vi "demark PXI-8431.vi"(8 "error In":errorcluster, 10 "Slot":i32=6) -> (0 "error out":errorcluster, 1 "COM name":string[](array[string]), 2 "VISA Ref":refnum<visa-resource-name>[](array[refnum]))   [LabVIEW 2017]
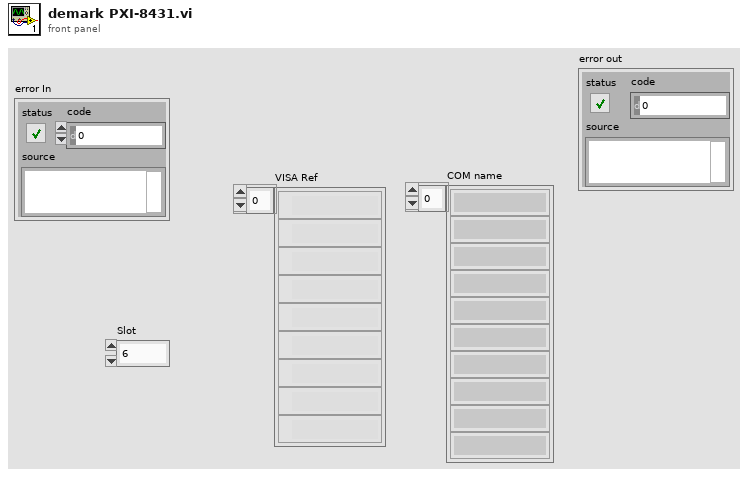
[diagram p1: front panel]
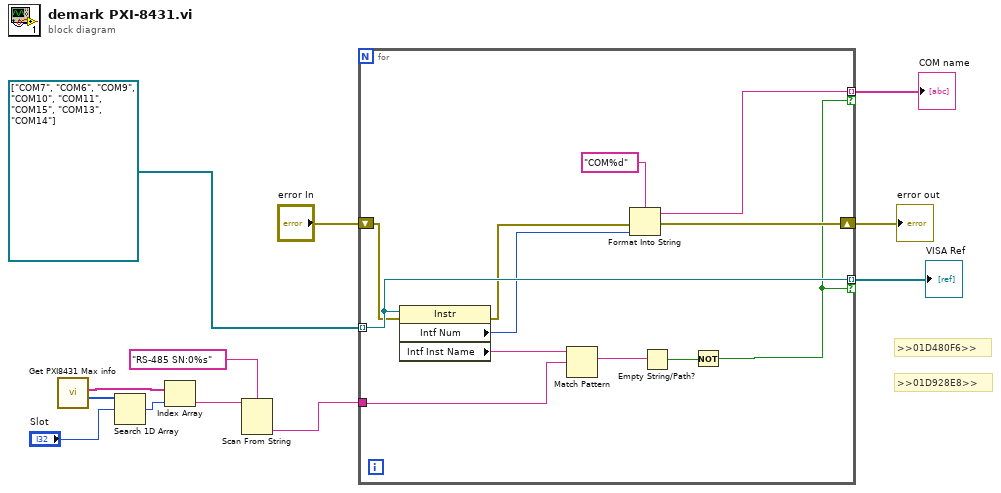
[diagram p0: block diagram]
diagram:
  # ">>01D480F6>>"
  # ">>01D928E8>>"
  n1 = call "Get PXI8431 Max info.vi"() -> ("Slot number"=w7:i32[], "Alias"=w5:string[])  [unwired: 10 in]
  n2 = Search 1D Array(1D array=w7, element="Slot") -> (index of element=w4:i32)  [unwired: 1 in]
  n3 = Index Array(array=w5, index=w4) -> (element=w3:string)
  n4 = Scan From String(format string="RS-485 SN:0%s", input string=w3) -> (output 1=w1:string)  [unwired: 3 in, 3 out]
  n5 = for {
    tunnel: refnum<visa-resource-name>[] ["COM7", "COM6", "COM9", "COM10", "COM11", "COM15", "COM13", "COM14"] -> [w24] mode=indexing
    tunnel: [w24] -> w11 mode=indexing if=w13
    tunnel: [w20] -> w8 mode=indexing if=w13
    shift-right: [w22] -> w9
    shift-left: "error In" -> [w21]
    tunnel: w1 -> [w16]
    n6 = property class="Instr"(reference=w24, error in=w21) -> (error out=w18:errorcluster, "Intf Num"=w19:u16, "Intf Inst Name"=w17:string)  [unwired: 1 out]
    n7 = Match Pattern(string=w17, regular expression=w16) -> (match substring=w15:string)  [unwired: 1 in, 3 out]
    n8 = Format Into String(format string="COM%d", error in=w18, w19) -> (resulting string=w20:string, error out=w22:errorcluster)  [unwired: 1 in]
    n9 = Empty String/Path?(string/path=w15) -> (empty?=w14:bool)
    n10 = Not(x=w14) -> (.not. x?=w13:bool)
  }
  "VISA Ref" <- w11
  "error out" <- w9
  "COM name" <- w8
